vi "TM open msg.vi"(8 "error in (no error)":errorcluster, 9 "timeout ms (1000)":i32=1000, 10 "Connected":bool, 11 "Queue in":T1) -> (0 "error out":errorcluster, 1 "timed out?":bool, 2 "Data":variant, 3 "Command":T2, 4 "Mailbox name":string, 5 "Unread":i32)   [LabVIEW 2021, in "Temperature monitor.lvlib"]
uses:
  Temperature monitor.lvlib
  <userlib>/MatS Libs/MatS Mailman/TypeDefs/Mailbox ref.ctl
  Typedefs/TM_commands.ctl
  <userlib>/MatS Libs/MatS Libs.lvlib
panel:
  out "mailbox ref out":T1
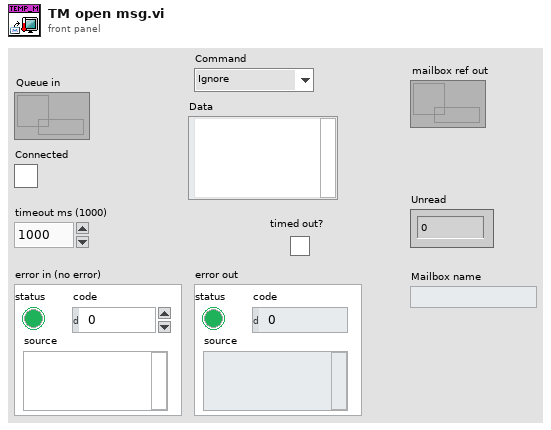
[diagram p1: front panel]
types:
  T1 = typedef "MatS Libs.lvlib/Mailbox ref.ctl" = refnum<queue>
  T2 = typedef "Temperature monitor.lvlib/TM_commands.ctl" = enum16{"Ignore", "Log", "Connect", "Set timeout", "Update", "Disconnect", "End"}
  T3 = typedef "MatS Libs.lvlib/General message.ctl" = cluster{"Sender":string, "Recipient":string, "Topic":variant, "Content":variant, "Time Stamp":timestamp}
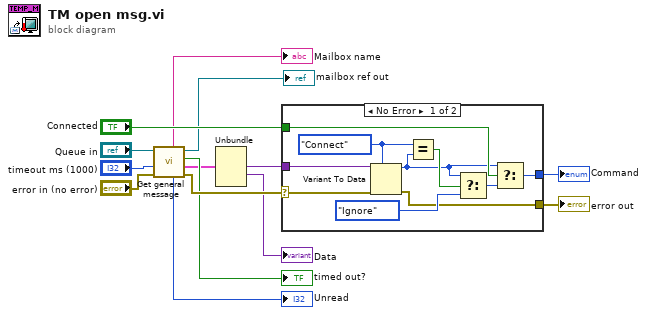
[diagram p0: block diagram]
diagram:
  n1 = call <userlib>:"Get general message.vi"("error in (no error)"="error in (no error)", "timeout ms (1000)"="timeout ms (1000)", "Mailbox ref in"="Queue in") -> ("error out"=w10:errorcluster, "Message"=w5:T3, "timed out?"=→"timed out?":bool, "mailbox ref out"=→"mailbox ref out":T1, "pending messages"=→"Unread":i32, "Mailbox name"=→"Mailbox name":string)  [unwired: 3 in]
  n2 = Unbundle(w5) -> ("Topic"=w2:variant, "Content"=→"Data":variant)  [unwired: 3 out]
  n3 = case shown="No Error" w10 {
    selector: w10 -> [w18 w25]
    tunnel: [w17 w25] -> w8
    tunnel: "Connected" -> [w24 _]
    tunnel: w2 -> [w20 _]
    tunnel: [w19 _] -> w7
    frame No Error {
      w15 = TM_commands."Connect" ("Command")
      n4 = Variant To Data(error in=w18, type=w15, Variant=w20) -> (data=w16:T2, error out=w17:errorcluster)
      n5 = Equal?(x=w15, y=w16) -> (x = y?=w23:bool)
      n6 = Select(t=w16, s=w23, f=TM_commands."Ignore" ("Command")) -> (s? t:f=w22:T2)
      n7 = Select(t=w16, s=w24, f=w22) -> (s? t:f=w19:T2)
    }
    frame Error {
    }
  }
  "error out" <- w8
  "Command" <- w7
